vi "Kiwi_Set_Output.vi"(8 "Rotation":dbl, 9 "Y":dbl, 10 "X":dbl, 11 "MotorDevRefs":T1={"Motor A"={"DeviceStatus"={"status"=FALSE, "code"=0, "source"=""}, "Type"=enum."PWM", "PWM"={"PWM Channel"=enum."Invalid", "DeadBand"={"Name"="", "maxPositivePwm"=0, "minPositivePwm"=0, "centerPwm"=0, "maxNegativePwm"=0, "minNegativePwm"=0, "angularRange"=0}}, "CAN"={"Device Number"=0, "SetOutput VI Ref"=variant(enum8{"Percent VBus", "Current", "Speed", "Position", "Voltage"} enum."Percent VBus"), "GetOutput VI Ref"=variant(refnum<k1> refnum), "Enable VI Ref"=variant(dbl 12.0), "Disable VI Ref"=variant(enum8{"Percent VBus", "Speed", "Position", "Slave", "Unchanged / Invalid", "Voltage Compensation", "Current", "Motion Profile"} enum."Percent VBus"), "Data"=variant}, "Invert"=FALSE}, "Motor B"={"DeviceStatus"={"status"=FALSE, "code"=0, "source"=""}, "Type"=enum."PWM", "PWM"={"PWM Channel"=enum."Invalid", "DeadBand"={"Name"="", "maxPositivePwm"=0, "minPositivePwm"=0, "centerPwm"=0, "maxNegativePwm"=0, "minNegativePwm"=0, "angularRange"=0}}, "CAN"={"Device Number"=0, "SetOutput VI Ref"=variant(enum8{"Percent VBus", "Current", "Speed", "Position", "Voltage"} enum."Percent VBus"), "GetOutput VI Ref"=variant(refnum<k1> refnum), "Enable VI Ref"=variant(dbl 12.0), "Disable VI Ref"=variant(enum8{"Percent VBus", "Speed", "Position", "Slave", "Unchanged / Invalid", "Voltage Compensation", "Current", "Motion Profile"} enum."Percent VBus"), "Data"=variant}, "Invert"=FALSE}, "Motor C"={"DeviceStatus"={"status"=FALSE, "code"=0, "source"=""}, "Type"=enum."PWM", "PWM"={"PWM Channel"=enum."Invalid", "DeadBand"={"Name"="", "maxPositivePwm"=0, "minPositivePwm"=0, "centerPwm"=0, "maxNegativePwm"=0, "minNegativePwm"=0, "angularRange"=0}}, "CAN"={"Device Number"=0, "SetOutput VI Ref"=variant(enum8{"Percent VBus", "Current", "Speed", "Position", "Voltage"} enum."Percent VBus"), "GetOutput VI Ref"=variant(refnum<k1> refnum), "Enable VI Ref"=variant(dbl 12.0), "Disable VI Ref"=variant(enum8{"Percent VBus", "Speed", "Position", "Slave", "Unchanged / Invalid", "Voltage Compensation", "Current", "Motion Profile"} enum."Percent VBus"), "Data"=variant}, "Invert"=FALSE}, "Config Consts"={"Arx"=0.0, "Ay"=0.0, "Brx"=0.0, "By"=0.0, "Cr"=0.0, "Cy"=0.0, "Cx"=0.0}, "status"={"status"=FALSE, "code"=0, "source"=""}, "Angles"={"Angle A"=60.0, "Angle B"=60.0, "Angle C"=60.0, "Radians?"=FALSE}, "MotorVals"={"MotorA"=0.0, "MotorB"=0.0, "MotorC"=0.0}}) -> (3 "MotorDevRefOut":T1={"Motor A"={"DeviceStatus"={"status"=FALSE, "code"=0, "source"=""}, "Type"=enum."PWM", "PWM"={"PWM Channel"=enum."Invalid", "DeadBand"={"Name"="", "maxPositivePwm"=0, "minPositivePwm"=0, "centerPwm"=0, "maxNegativePwm"=0, "minNegativePwm"=0, "angularRange"=0}}, "CAN"={"Device Number"=0, "SetOutput VI Ref"=variant(enum8{"Percent VBus", "Current", "Speed", "Position", "Voltage"} enum."Percent VBus"), "GetOutput VI Ref"=variant(refnum<k1> refnum), "Enable VI Ref"=variant(dbl 12.0), "Disable VI Ref"=variant(enum8{"Percent VBus", "Speed", "Position", "Slave", "Unchanged / Invalid", "Voltage Compensation", "Current", "Motion Profile"} enum."Percent VBus"), "Data"=variant}, "Invert"=FALSE}, "Motor B"={"DeviceStatus"={"status"=FALSE, "code"=0, "source"=""}, "Type"=enum."PWM", "PWM"={"PWM Channel"=enum."Invalid", "DeadBand"={"Name"="", "maxPositivePwm"=0, "minPositivePwm"=0, "centerPwm"=0, "maxNegativePwm"=0, "minNegativePwm"=0, "angularRange"=0}}, "CAN"={"Device Number"=0, "SetOutput VI Ref"=variant(enum8{"Percent VBus", "Current", "Speed", "Position", "Voltage"} enum."Percent VBus"), "GetOutput VI Ref"=variant(refnum<k1> refnum), "Enable VI Ref"=variant(dbl 12.0), "Disable VI Ref"=variant(enum8{"Percent VBus", "Speed", "Position", "Slave", "Unchanged / Invalid", "Voltage Compensation", "Current", "Motion Profile"} enum."Percent VBus"), "Data"=variant}, "Invert"=FALSE}, "Motor C"={"DeviceStatus"={"status"=FALSE, "code"=0, "source"=""}, "Type"=enum."PWM", "PWM"={"PWM Channel"=enum."Invalid", "DeadBand"={"Name"="", "maxPositivePwm"=0, "minPositivePwm"=0, "centerPwm"=0, "maxNegativePwm"=0, "minNegativePwm"=0, "angularRange"=0}}, "CAN"={"Device Number"=0, "SetOutput VI Ref"=variant(enum8{"Percent VBus", "Current", "Speed", "Position", "Voltage"} enum."Percent VBus"), "GetOutput VI Ref"=variant(refnum<k1> refnum), "Enable VI Ref"=variant(dbl 12.0), "Disable VI Ref"=variant(enum8{"Percent VBus", "Speed", "Position", "Slave", "Unchanged / Invalid", "Voltage Compensation", "Current", "Motion Profile"} enum."Percent VBus"), "Data"=variant}, "Invert"=FALSE}, "Config Consts"={"Arx"=0.0, "Ay"=0.0, "Brx"=0.0, "By"=0.0, "Cr"=0.0, "Cy"=0.0, "Cx"=0.0}, "status"={"status"=FALSE, "code"=0, "source"=""}, "Angles"={"Angle A"=60.0, "Angle B"=60.0, "Angle C"=60.0, "Radians?"=FALSE}, "MotorVals"={"MotorA"=0.0, "MotorB"=0.0, "MotorC"=0.0}})   [LabVIEW 2016]
uses:
  <userlib>/836-Libraries/Drive/kiwi/support/Kiwi_Dev_Ref.ctl
  <vilib>/Rock Robotics/WPI/MotorControl/WPI_MotorControlDeviceRef.ctl
  <vilib>/Rock Robotics/WPI/MotorControl/WPI_MotorControlType.ctl
  <vilib>/Rock Robotics/SystemInterfaces/DIO/FPGA_DIOPWMChannel.ctl
  <vilib>/Rock Robotics/WPI/PWM/WPI_PWMDeadband.ctl
  <userlib>/836-Libraries/Drive/kiwi/support/Kiwi_Cal_Constants.ctl
  <userlib>/836-Libraries/Drive/kiwi/support/Kiwi_Angles.ctl
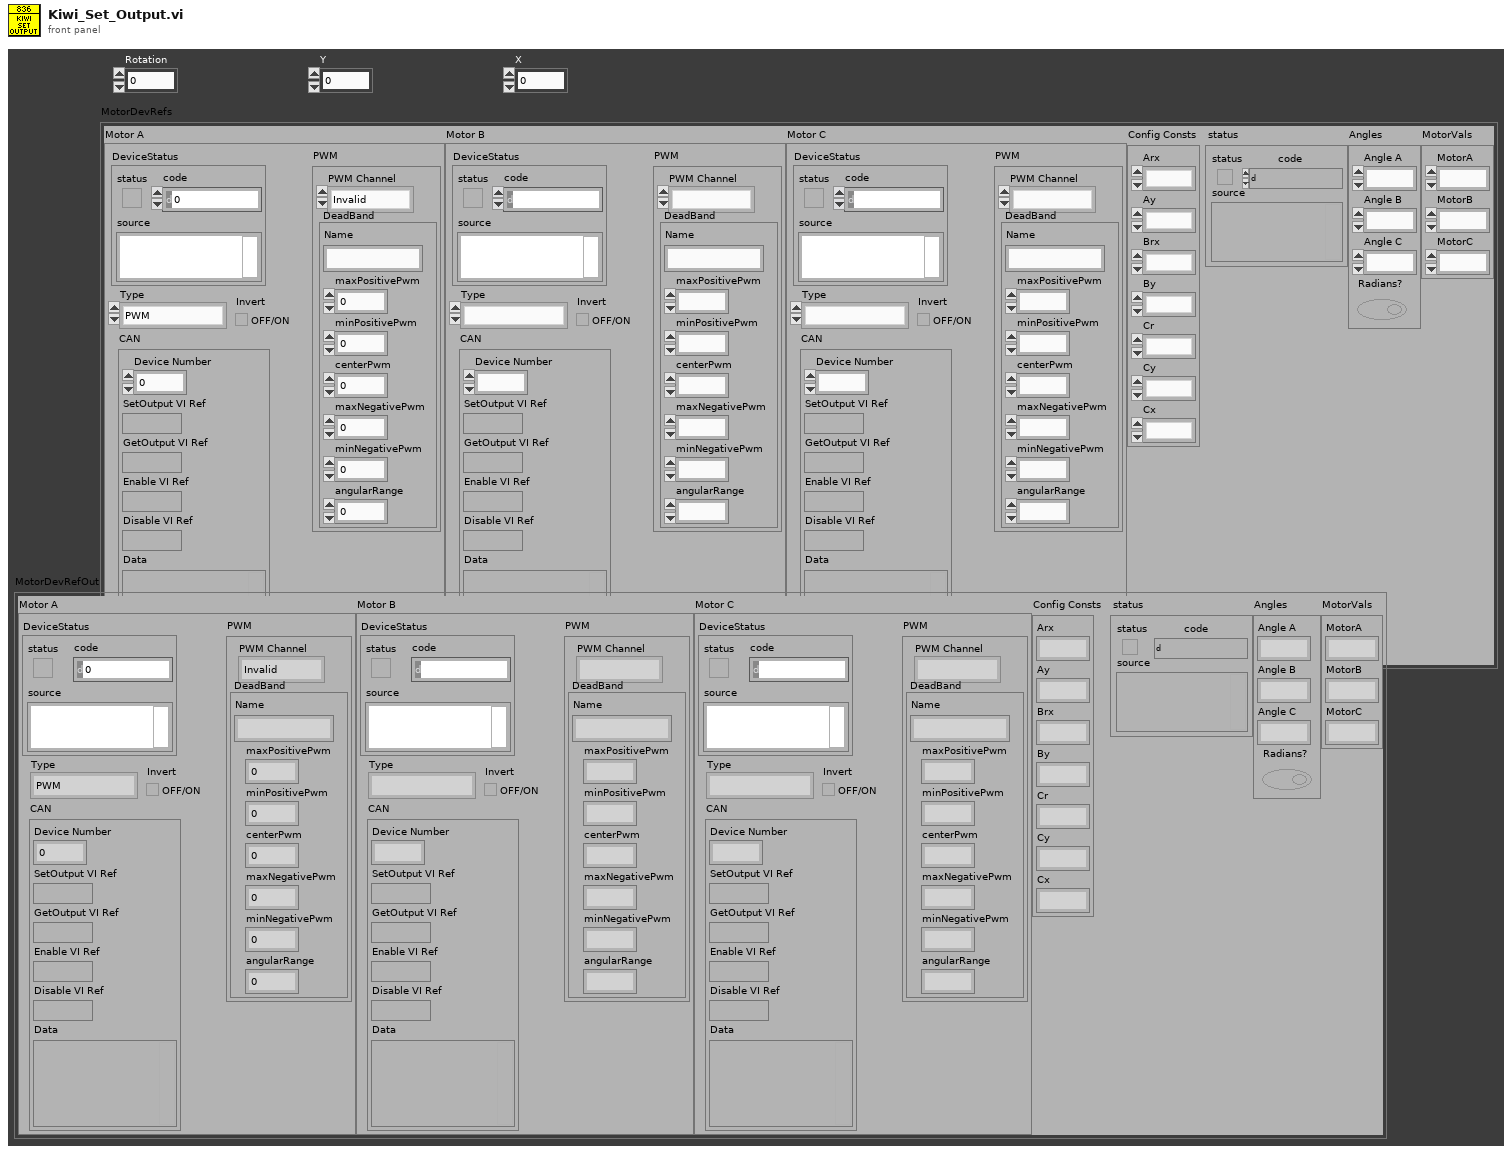
[diagram p1: front panel]
types:
  T1 = typedef "Kiwi_Dev_Ref.ctl" = cluster{"Motor A":T2, "Motor B":T2, "Motor C":T2, "Config Consts":T6, "status":errorcluster, "Angles":T7, "MotorVals":cluster{"MotorA":dbl, "MotorB":dbl, "MotorC":dbl}}
  T2 = typedef "WPI_MotorControlDeviceRef.ctl" = cluster{"DeviceStatus":errorcluster, "Type":T3, "PWM":cluster{"PWM Channel":T4, "DeadBand":T5}, "CAN":cluster{"Device Number":u8, "SetOutput VI Ref":variant, "GetOutput VI Ref":variant, "Enable VI Ref":variant, "Disable VI Ref":variant, "Data":variant}, "Invert":bool}
  T3 = typedef "WPI_MotorControlType.ctl" = enum16{"PWM", "CAN"}
  T4 = typedef "FPGA_DIOPWMChannel.ctl" = enum8{"PWM 0", "PWM 1", "PWM 2", "PWM 3", "PWM 4", "PWM 5", "PWM 6", "PWM 7", "PWM 8", "PWM 9", "PWM MXP 0", "PWM MXP 1", "PWM MXP 2", "PWM MXP 3", "PWM MXP 4", "PWM MXP 5", "PWM MXP 6", "PWM MXP 7", "PWM MXP 8", "PWM MXP 9", "Invalid"}
  T5 = typedef "WPI_PWMDeadband.ctl" = cluster{"Name":string, "maxPositivePwm":i32, "minPositivePwm":i32, "centerPwm":i32, "maxNegativePwm":i32, "minNegativePwm":i32, "angularRange":u16}
  T6 = typedef "Kiwi_Cal_Constants.ctl" = cluster{"Arx":dbl, "Ay":dbl, "Brx":dbl, "By":dbl, "Cr":dbl, "Cy":dbl, "Cx":dbl}
  T7 = typedef "Kiwi_Angles.ctl" = cluster{"Angle A":dbl, "Angle B":dbl, "Angle C":dbl, "Radians?":bool}
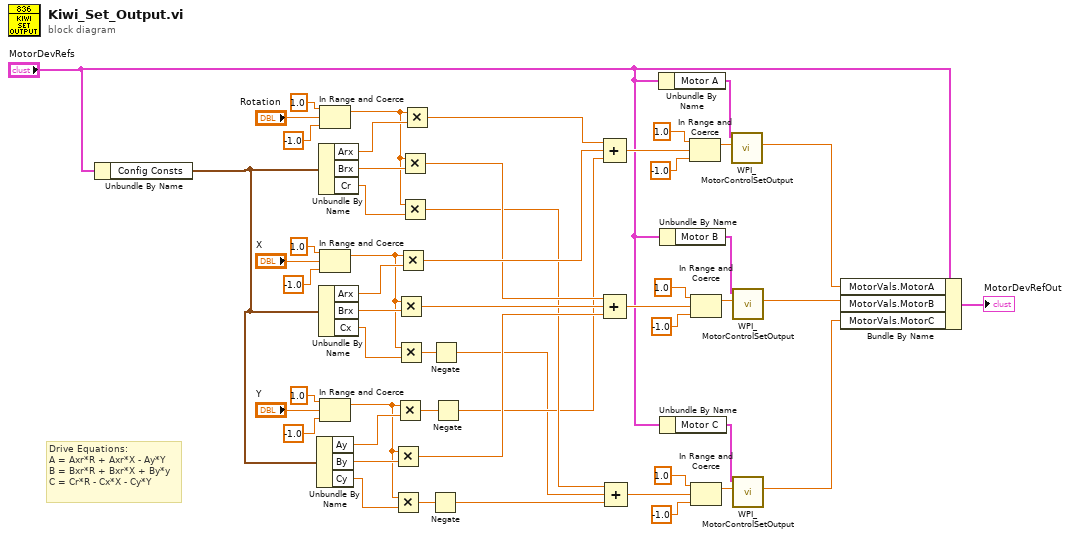
[diagram p0: block diagram]
diagram:
  # "Drive Equations:\nA = Axr*R + Axr*X - Ay*Y\nB = Bxr*R + Bxr*X + By*y\nC = Cr*R - Cx*X - Cy*Y"
  n1 = Unbundle By Name("MotorDevRefs") -> ("Config Consts"=w5:T6)
  n2 = Unbundle By Name(w5) -> ("Ay"=w42:dbl, "By"=w43:dbl, "Cy"=w44:dbl)
  n3 = Unbundle By Name(w5) -> ("Arx"=w47:dbl, "Brx"=w46:dbl, "Cr"=w45:dbl)
  n4 = Unbundle By Name(w5) -> ("Arx"=w50:dbl, "Brx"=w49:dbl, "Cx"=w48:dbl)
  n5 = In Range and Coerce(upper limit=1.0, x="Rotation", lower limit=-1.0) -> (coerced(x)=w13:dbl)  [unwired: 1 out]
  n6 = In Range and Coerce(upper limit=1.0, x="X", lower limit=-1.0) -> (coerced(x)=w17:dbl)  [unwired: 1 out]
  n7 = In Range and Coerce(upper limit=1.0, x="Y", lower limit=-1.0) -> (coerced(x)=w19:dbl)  [unwired: 1 out]
  n8 = Multiply(x=w19, y=w43) -> (x*y=w36:dbl)
  n9 = Multiply(x=w19, y=w44) -> (x*y=w35:dbl)
  n10 = Multiply(x=w19, y=w42) -> (x*y=w39:dbl)
  n11 = Multiply(x=w17, y=w49) -> (x*y=w37:dbl)
  n12 = Multiply(x=w17, y=w48) -> (x*y=w4:dbl)
  n13 = Multiply(x=w17, y=w50) -> (x*y=w40:dbl)
  n14 = Multiply(x=w13, y=w46) -> (x*y=w38:dbl)
  n15 = Multiply(x=w13, y=w45) -> (x*y=w34:dbl)
  n16 = Multiply(x=w13, y=w47) -> (x*y=w41:dbl)
  n17 = Negate(x=w35) -> (-x=w1:dbl)
  n18 = Negate(x=w4) -> (-x=w2:dbl)
  n19 = Negate(x=w39) -> (-x=w3:dbl)
  n20 = Compound Arithmetic op=ADD(w41, w40, w3) -> (w24:dbl)
  n21 = Compound Arithmetic op=ADD(w38, w37, w36) -> (w23:dbl)
  n22 = Compound Arithmetic op=ADD(w34, w2, w1) -> (w33:dbl)
  n23 = Unbundle By Name("MotorDevRefs") -> ("Motor A"=w25:T2)
  n24 = Unbundle By Name("MotorDevRefs") -> ("Motor B"=w29:T2)
  n25 = Unbundle By Name("MotorDevRefs") -> ("Motor C"=w51:T2)
  n26 = In Range and Coerce(upper limit=1.0, x=w24, lower limit=-1.0) -> (coerced(x)=w26:dbl)  [unwired: 1 out]
  n27 = In Range and Coerce(upper limit=1.0, x=w23, lower limit=-1.0) -> (coerced(x)=w30:dbl)  [unwired: 1 out]
  n28 = In Range and Coerce(upper limit=1.0, x=w33, lower limit=-1.0) -> (coerced(x)=w52:dbl)  [unwired: 1 out]
  n29 = call <vilib>:"WPI_MotorControlSetOutput.vi"("Output"=w26, "MotorControlDevRef"=w25) -> ("Motor Output"=w8:dbl)  [unwired: 7 in, 2 out]
  n30 = call <vilib>:"WPI_MotorControlSetOutput.vi"("Output"=w30, "MotorControlDevRef"=w29) -> ("Motor Output"=w7:dbl)  [unwired: 7 in, 2 out]
  n31 = call <vilib>:"WPI_MotorControlSetOutput.vi"("Output"=w52, "MotorControlDevRef"=w51) -> ("Motor Output"=w6:dbl)  [unwired: 7 in, 2 out]
  n32 = Bundle By Name(cluster="MotorDevRefs", "MotorVals.MotorA"=w8, "MotorVals.MotorB"=w7, "MotorVals.MotorC"=w6) -> (→"MotorDevRefOut":T1)
